vi "fisiere_v1.vi"() -> ()   [LabVIEW 2009]
panel:
  out "Citire din fisier terminata":bool
  out "Tari si capitale":string[](array[string])
  in  "Selectati calea si fisierul":path=path "E:/Projects/Lab_view/Vi/fisiere/country-capital.txt"
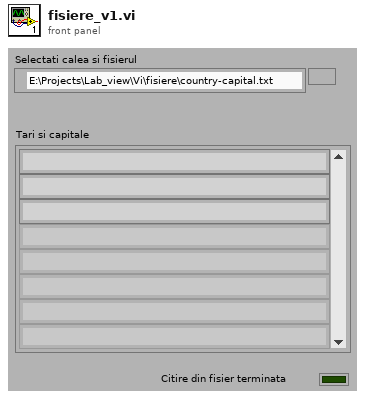
[diagram p1: front panel]
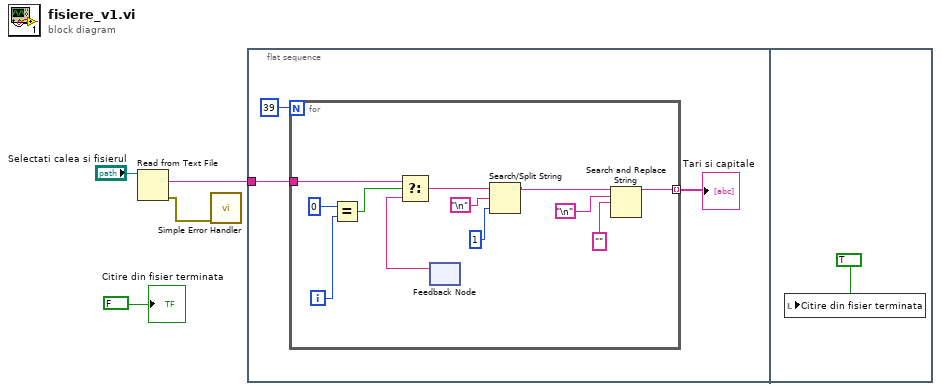
[diagram p0: block diagram]
diagram:
  n1 = Read from Text File(file (use dialog)="Selectati calea si fisierul") -> (text=w3:string, error out=w2:errorcluster)  [unwired: 3 in, 2 out]
  n2 = call <vilib>:"Simple Error Handler.vi"("error in (no error)"=w2) -> ()  [unwired: 4 in, 5 out]
  n3 = flat-sequence {
    tunnel: w3 -> [w7]
    frame #0 {
      n4 = for {
        N: 39 -> [_]
        tunnel: w7 -> [w17]
        tunnel: [w8] -> w5 mode=indexing
        i -> [w16]
        n5 = Equal?(x=0, y=w16) -> (x = y?=w14:bool)
        n6 = feedback #1() -> (w18:string)  [unwired: 1 in]
        n7 = Select(t=w17, s=w14, f=w18) -> (s? t:f=w13:string)
        n8 = Search/Split String(string=w13, search string/char (-)="\n", offset (0)=1) -> (substring before match=w9:string, match + rest of string=w12:string)  [unwired: 1 out]
        n9 = Search and Replace String(input string=w9, search string="\n", replace string="") -> (result string=w8:string)  [unwired: 5 in, 3 out]
      }
      "Tari si capitale" <- w5
    }
    frame #1 {
      n10 = local write "Citire din fisier terminata"(TRUE ("Ready")) -> ()
    }
  }
  "Citire din fisier terminata" <- FALSE ("Af_start")
